vi "Process Mouse Move.vi"(0 "State":T1={"Nspeakers"=13, "actions"=[], "Wspeaker"=13, "Wmic"=13, "sel mic"=13, "hover"={"type"=enum."None", "index"=0}, "locked"=FALSE, "states"=[], "sel speak"=13, "selected"=refnum, "Events"={"Mic change"=refnum, "Selection change"=refnum}}, 5 "Layout":T6, 7 "Coords":T8) -> (8 "Hover Data":T2)   [LabVIEW 2015, in "HRTF Config.xctl"]
uses:
  HRTF Config.xctl
  <vilib>/Utility/miscctls.llb/LVPoint32TypeDef.ctl
  Layout.ctl
  Item.ctl
  Hover Data.ctl
  Hover Item.ctl
  State.vi
  Speaker State.ctl
  Events.ctl
  Selection changed.ctl
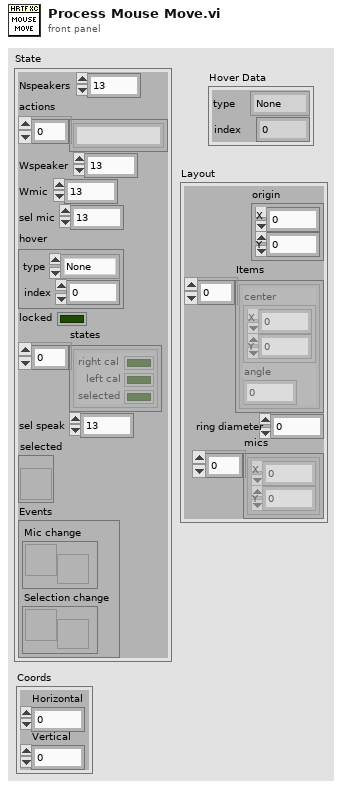
[diagram p1: front panel]
types:
  T1 = typedef "HRTF Config.xctl/State.vi" = cluster{"Nspeakers":i32, "actions":string[], "Wspeaker":i32, "Wmic":i32, "sel mic":i32, "hover":T2, "locked":bool, "states":T4[], "sel speak":i32, "selected":refnum<vi>, "Events":T5}
  T2 = typedef "HRTF Config.xctl/Hover Data.ctl" = cluster{"type":T3, "index":i32}
  T3 = typedef "HRTF Config.xctl/Hover Item.ctl" = enum16{"None", "Speaker", "Mic"}
  T4 = typedef "HRTF Config.xctl/Speaker State.ctl" = cluster{"right cal":bool, "left cal":bool, "selected":bool}
  T5 = typedef "HRTF Config.xctl/Events.ctl" = cluster{"Mic change":refnum<user-event>, "Selection change":refnum<user-event>}
  T6 = typedef "HRTF Config.xctl/Layout.ctl" = cluster{"origin":cluster{"X":i32, "Y":i32}, "Items":T7[], "ring diameter":i32, "mics":cluster{"X":i32, "Y":i32}[]}
  T7 = typedef "HRTF Config.xctl/Item.ctl" = cluster{"center":cluster{"X":i32, "Y":i32}, "angle":dbl}
  T8 = typedef "LVPoint32TypeDef.ctl" = cluster{"Horizontal":i32, "Vertical":i32}
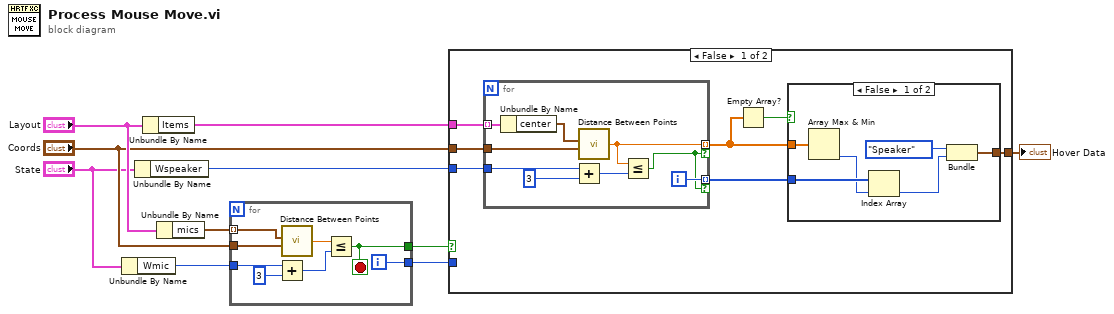
[diagram p0: block diagram]
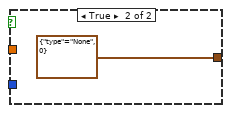
[diagram p2: hidden frame]
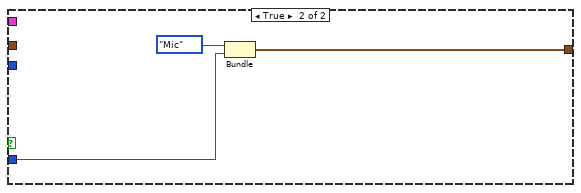
[diagram p3: hidden frame]
diagram:
  n1 = Unbundle By Name("State") -> ("Wmic"=w9:i32)
  n2 = Unbundle By Name("State") -> ("Wspeaker"=w1:i32)
  n3 = Unbundle By Name("Layout") -> ("Items"=w4:T7[])
  n4 = Unbundle By Name("Layout") -> ("mics"=w10:cluster{"X":i32, "Y":i32}[])
  n5 = for {
    tunnel: w10 -> [w18] mode=indexing
    tunnel: "Coords" -> [w17]
    tunnel: w9 -> [w15]
    tunnel: [w14] -> w8
    tunnel: [w13] -> w7
    i -> [w13]
    stop <- w14 stop-if-true
    n6 = Add(x=w15, y=3) -> (x+y=w12:i32)
    n7 = call "Distance Between Points.vi"("B"=w17, "A"=w18) -> ("distance"=w16:dbl)  [unwired: 4 in]
    n8 = Less Or Equal?(x=w16, y=w12) -> (x <= y?=w14:bool)
  }
  n9 = case shown="False" w8 {
    tunnel: w7 -> [_ w43]
    tunnel: [w25 w42] -> w6
    tunnel: w4 -> [w24 _]
    tunnel: "Coords" -> [w23 _]
    tunnel: w1 -> [w22 _]
    frame False {
      n10 = for {
        tunnel: w24 -> [w41] mode=indexing
        tunnel: w23 -> [w40]
        tunnel: w22 -> [w39]
        tunnel: [w38] -> w19 mode=indexing if=w33
        tunnel: [w34] -> w20 mode=indexing if=w33
        i -> [w38]
        n11 = Unbundle By Name(w41) -> ("center"=w35:cluster{"X":i32, "Y":i32})
        n12 = Add(x=w39, y=3) -> (x+y=w37:i32)
        n13 = call "Distance Between Points.vi"("B"=w40, "A"=w35) -> ("distance"=w34:dbl)  [unwired: 4 in]
        n14 = Less Or Equal?(x=w34, y=w37) -> (x <= y?=w33:bool)
      }
      n15 = Empty Array?(array=w20) -> (empty?=w21:bool)
      n16 = case shown="False" w21 {
        tunnel: [w30 cluster{"type":T3, i32} {"type"=enum."None", 0}] -> w25
        tunnel: w20 -> [w29 _]
        tunnel: w19 -> [w28 _]
        frame False {
          n17 = Array Max & Min(array=w29) -> (min index (indices)=w27:i32)  [unwired: 3 out]
          n18 = Index Array(array=w28, index=w27) -> (element=w26:i32)
          n19 = Bundle("type"=Hover_Item."Speaker", w26) -> (w30:cluster{"type":T3, i32})  [unwired: 1 in]
        }
        frame True {
        }
      }
    }
    frame True {
      n20 = Bundle("type"=Hover_Item."Mic", w43) -> (w42:cluster{"type":T3, i32})  [unwired: 1 in]
    }
  }
  "Hover Data" <- w6
